vi "MTM2_waitForCompletion_clearErrors.vi"(8 "error in (no error)":errorcluster, 11 "waitComplete_Ctl":T1) -> (0 "error out":errorcluster, 2 "function return":i32, 3 "waitComplete_Ctl out":T1)   [LabVIEW 2018, in "SALLV_MTM2.lvlib"]
doc: "int MTM2_shm_waitForCompletion_clearErrorsLV(MTM2_waitCompleteLV *waitComplete_Ctl);"
uses:
  SALLV_MTM2.lvlib
  SALLV_MTM2.so
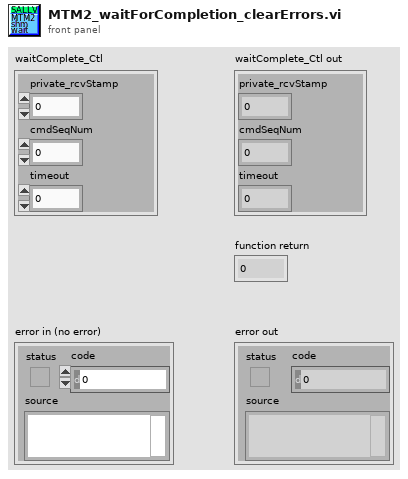
[diagram p1: front panel]
types:
  T1 = cluster{"private_rcvStamp":dbl, "cmdSeqNum":i32, "timeout":u32}
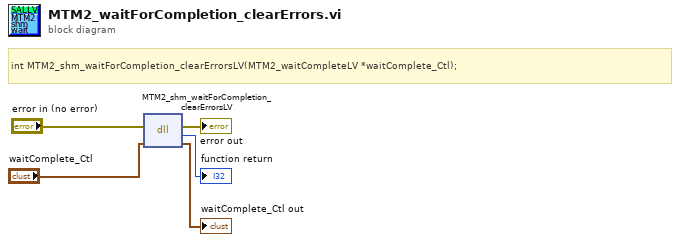
[diagram p0: block diagram]
diagram:
  # "int MTM2_shm_waitForCompletion_clearErrorsLV(MTM2_waitCompleteLV *waitComplete_Ctl);"
  n1 = dll-call lib="home/ttsai/Documents/salTestLabViewApi/SALLV_MTM2/SALLV_MTM2.*" fn="MTM2_shm_waitForCompletion_clearErrorsLV"(error in="error in (no error)", "waitComplete_Ctl"="waitComplete_Ctl") -> (error out=→"error out":errorcluster, →"function return":i32, "waitComplete_Ctl"=→"waitComplete_Ctl out":T1)  [unwired: 2 in, 1 out]
